vi "Clear Self.vi"(8 "error in (no error)":errorcluster, 10 "Picture in":picture, 11 "Polygon in":refnum<class "Polygon.lvclass">) -> (0 "error out":errorcluster, 2 "Picture out":picture, 3 "Polygon out":refnum<class "Polygon.lvclass">)   [LabVIEW 2015, in "Polygon.lvclass"]
uses:
  Polygon.lvclass
  Polygon.lvclass/Polygon.ctl
  Line/Line.lvclass
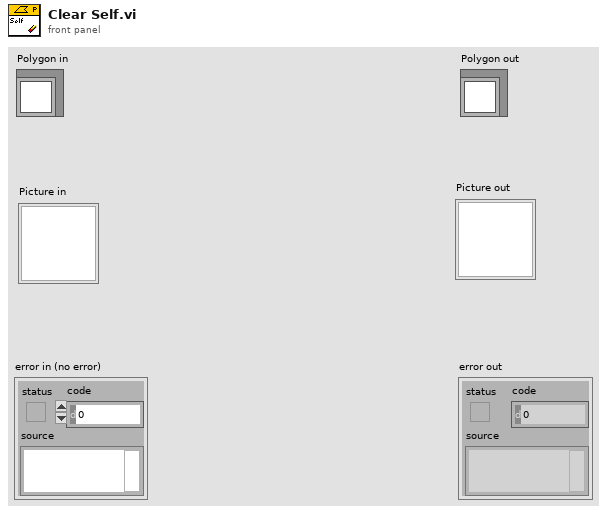
[diagram p1: front panel]
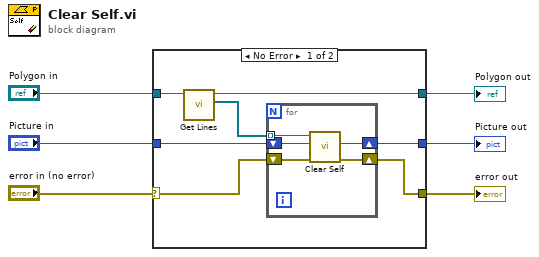
[diagram p0: block diagram]
diagram:
  n1 = case shown="No Error" "error in (no error)" {
    selector: "error in (no error)" -> [w8 w21]
    tunnel: "Polygon in" -> [w13 w20]
    tunnel: [w12 w20] -> w5
    tunnel: "Picture in" -> [w11 w19]
    tunnel: [w9 w19] -> w2
    tunnel: [w7 w21] -> w1
    frame No Error {
      n2 = call "Get Lines.vi"("Polygon in"=w13) -> ("Lines"=w10:refnum<class "Line.lvclass">[], "Polygon out"=w12:refnum<class "Polygon.lvclass">)  [unwired: 8 in, 1 out]
      n3 = for {
        shift-right: [w17] -> w9
        shift-left: w11 -> [w18]
        tunnel: w10 -> [w16] mode=indexing
        shift-right: [w14] -> w7
        shift-left: w8 -> [w15]
        n4 = call-dynamic "Clear Self.vi"("error in (no error)"=w15, "Picture in"=w18, "Line in"=w16) -> ("error out"=w14:errorcluster, "Picture out"=w17:picture)  [unwired: 6 in, 1 out]
      }
    }
    frame Error {
    }
  }
  "error out" <- w1
  "Polygon out" <- w5
  "Picture out" <- w2
